vi "SVs_Variable1.vi"() -> ()   [LabVIEW 2010]
panel:
  in  "SVs_Variable1":dbl
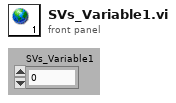
[diagram p1: front panel]
diagram:
